vi "produce data.vi"() -> (3 "res":string[][](array[string]))   [LabVIEW 2018]
uses:
  PC/class/pyCode/pyCode.lvclass
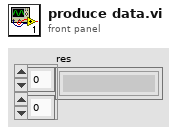
[diagram p1: front panel]
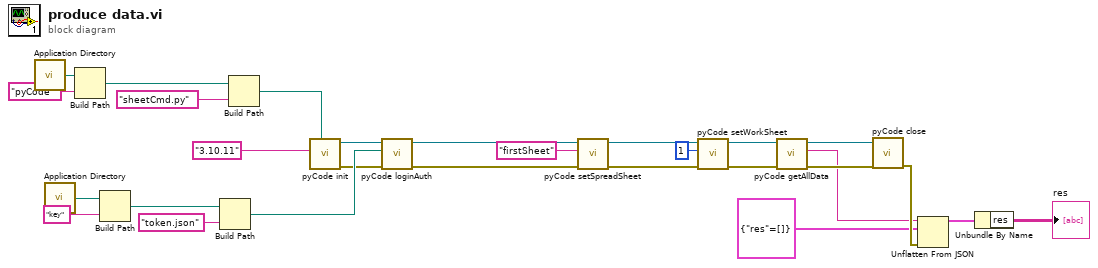
[diagram p0: block diagram]
diagram:
  n1 = call <vilib>:"Application Directory.vi"() -> ("Application Directory"=w11:path)
  n2 = call <vilib>:"Application Directory.vi"() -> ("Application Directory"=w12:path)
  n3 = Build Path(base path=w11, name or relative path="pyCode") -> (appended path=w10:path)
  n4 = Build Path(base path=w12, name or relative path="key") -> (appended path=w13:path)
  n5 = Build Path(base path=w13, name or relative path="token.json") -> (appended path=w16:path)
  n6 = Build Path(base path=w10, name or relative path="sheetCmd.py") -> (appended path=w17:path)
  n7 = call "pyCode init.vi"("pyCmdFilePath"=w17, "pyVersion"="3.10.11" ("Python version")) -> ("error out"=w15:errorcluster, "pyCode out"=w14:refnum<class "pyCode.lvclass">)  [unwired: 8 in]
  n8 = call "pyCode loginAuth.vi"("error in (no error)"=w15, "tokenFilePath"=w16, "pyCode in"=w14) -> ("error out"=w19:errorcluster, "pyCode out"=w18:refnum<class "pyCode.lvclass">)  [unwired: 7 in]
  n9 = call "pyCode setSpreadSheet.vi"("error in (no error)"=w19, "sheetName"="firstSheet", "pyCode in"=w18) -> ("error out"=w20:errorcluster, "pyCode out"=w21:refnum<class "pyCode.lvclass">)  [unwired: 7 in]
  n10 = call "pyCode setWorkSheet.vi"("error in (no error)"=w20, "idx"=1, "pyCode in"=w21) -> ("error out"=w24:errorcluster, "pyCode out"=w23:refnum<class "pyCode.lvclass">)  [unwired: 7 in]
  n11 = call "pyCode getAllData.vi"("error in (no error)"=w24, "pyCode in"=w23) -> ("error out"=w27:errorcluster, "response"=w22:string, "pyCode out"=w26:refnum<class "pyCode.lvclass">)  [unwired: 7 in]
  n12 = call "pyCode close.vi"("error in (no error)"=w27, "pyCode in"=w26) -> ("error out"=w28:errorcluster)  [unwired: 8 in, 1 out]
  n13 = Unflatten From JSON(JSON string=w22, type and defaults=cluster{"res":string[][]} {"res"=[]}, error in (no error)=w28) -> (value=w25:cluster{"res":string[][]})  [unwired: 4 in, 1 out]
  n14 = Unbundle By Name(w25) -> ("res"=→"res":string[][])
